vi "Write--command.vi"(8 "error in (no error)":errorcluster, 10 "Command":string, 11 "VISA resource name":refnum<visa-resource-name>) -> (0 "error out":errorcluster, 2 "Command out":string, 3 "VISA resource name out":refnum<visa-resource-name>)   [LabVIEW 2025, in "Control de MaP.lvlib"]
doc: "convierte la selección de comando a cadena y lo envía al puerto seleccionado"
uses:
  Control de MaP.lvlib
  <vilib>/Instr/_visa.llb/VISA Flush IO Buffer Mask.ctl
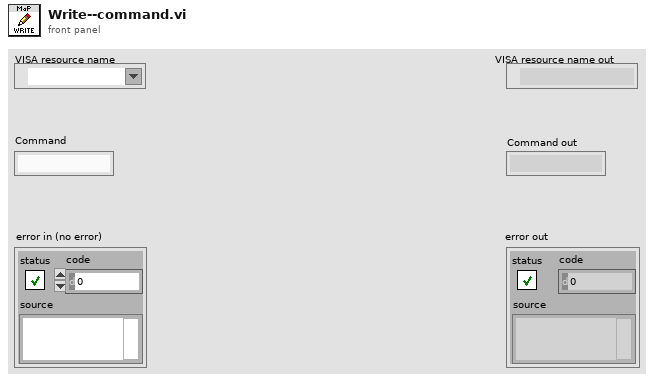
[diagram p1: front panel]
types:
  T1 = typedef "VISA Flush IO Buffer Mask.ctl" = u16
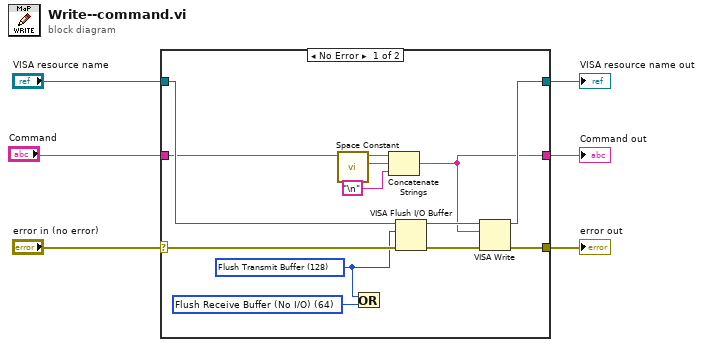
[diagram p0: block diagram]
diagram:
  n1 = case shown="No Error" "error in (no error)" {
    selector: "error in (no error)" -> [w15 w20]
    tunnel: "VISA resource name" -> [w14 w19]
    tunnel: [w18 w19] -> w5
    tunnel: [w17 w20] -> w3
    tunnel: "Command" -> [w10 _]
    tunnel: [w7 _] -> w1
    frame No Error {
      w16 = T1 64 items=["Flush Receive Buffer"=16, "Write Transmit Buffer to Device"=32, "Flush Receive Buffer (No I/O)"=64, "Flush Transmit Buffer"=128] ("Mask")
      w11 = T1 128 items=["Flush Receive Buffer"=16, "Write Transmit Buffer to Device"=32, "Flush Receive Buffer (No I/O)"=64, "Flush Transmit Buffer"=128] ("Mask")
      n2 = call <vilib>:"Space Constant.vi"() -> ("String"=w9:string)
      n3 = Or(x=w11, y=w16) -> ()  [unwired: 1 out]
      n4 = Concatenate Strings(w10, w9, "\n") -> (w7:string)
      n5 = VISA Flush I/O Buffer(VISA resource name=w14, mask (16)=w11, error in (no error)=w15) -> (VISA resource name out=w13:refnum<visa-resource-name>, error out=w12:errorcluster)
      n6 = VISA Write(VISA resource name=w13, write buffer=w7, error in (no error)=w12) -> (VISA resource name out=w18:refnum<visa-resource-name>, error out=w17:errorcluster)  [unwired: 1 out]
    }
    frame Error {
    }
  }
  "VISA resource name out" <- w5
  "error out" <- w3
  "Command out" <- w1
